vi "Measurement Logic.vi"() -> ()   [LabVIEW 2024, in "Analog Tachometer.lvlib"]
uses:
  Analog Tachometer.lvlib
  <vilib>/Plug-In SDKs/Measurements/Measure Call Context/Measure Call Context.lvclass
  Measurement Results.ctl
  <vilib>/gRPC/Generated APIs/ni/protobuf/types/RPC Messages/ni_protobuf_types_DoubleXYData.ctl
  <extravilib>/ChannelInstances/Event Messenger-bool/Instantiate.vi
  <vilib>/gRPC/Generated APIs/ni/protobuf/types/ni.protobuf.types.lvlib
  <vilib>/addons/Sound and Vibration/Order Analysis/Tach Process/SoundVib_TachProcess.lvlib
  <vilib>/addons/Sound and Vibration/Order Analysis/Utility/SoundVib_OAUtility.lvlib
  <vilib>/addons/Sound and Vibration/Order Analysis/Utility/SubVIs/oa_Buffer Settings.ctl
  <resource>/objmgr/daqmx.rc
  <vilib>/addons/Sound and Vibration/Order Analysis/Utility/OAT Output Buffered Data (XY, 1 Chan).vi
  <vilib>/DAQmx/read.llb/DAQmx Read (Analog Wfm 1Chan NSamp).vi
  <vilib>/addons/Sound and Vibration/Order Analysis/Tach Process/OAT Analog Tacho Process (1 Tacho).vi
  <vilib>/DAQmx/create/channels.llb/DAQmx Create Channel (AI-Voltage-Basic).vi
  <vilib>/DAQmx/configure/timing.llb/DAQmx Timing (Sample Clock).vi
  Measurement Configuration.ctl
panel:
  out "measurement results":T1
  in  "measurement configuration":T3={"sample rate"=1.2, "channel"="Lorem ipsum dolor sit", "max voltage"=32.0, "IEPE current"=32.0, "coupling"=64, "pulse/rev"=64, "threshold"=-32.0, "hysteresis"=-32.0, "slope (Rising)"=0} {"slope (Rising)" items=["Rising", "Falling"]; "coupling" items=["AC"=10045, "DC"=10050, "GND"=10066]}
  out "measure call context out":refnum<class "Measure Call Context.lvclass">
  in  "measure call context in":refnum<class "Measure Call Context.lvclass">
  out "error out":errorcluster
  in  "error in":errorcluster
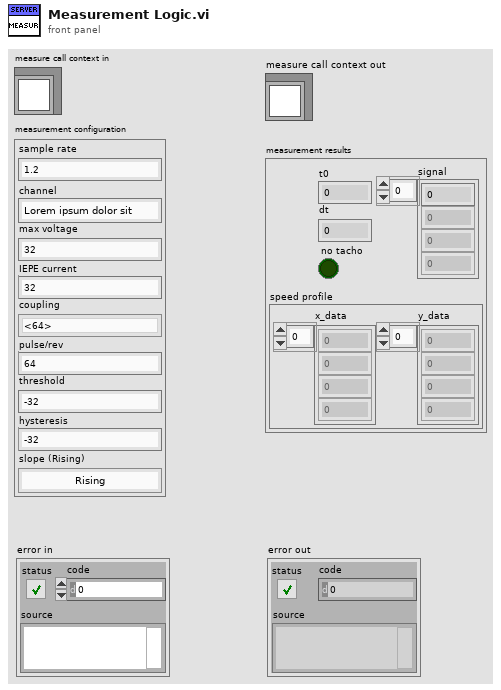
[diagram p1: front panel]
types:
  T1 = typedef "Analog Tachometer.lvlib/Measurement Results.ctl" = cluster{"t0":dbl, "dt":dbl, "signal":dbl[], "no tacho":bool, "speed profile":T2}
  T2 = typedef "ni.protobuf.types.lvlib/ni_protobuf_types_DoubleXYData.ctl" = cluster{"x_data":dbl[], "y_data":dbl[]}
  T3 = typedef "Analog Tachometer.lvlib/Measurement Configuration.ctl" = cluster{"sample rate":dbl, "channel":string, "max voltage":dbl, "IEPE current":dbl, "coupling":i32, "pulse/rev":i32, "threshold":dbl, "hysteresis":dbl, "slope (Rising)":u32}
  T4 = typedef "SoundVib_OAUtility.lvlib/oa_Buffer Settings.ctl" = cluster{"buffer size":dbl, "buffer unit":enum16{"s", "revolution", "# of samples"}}
  T5 = typedef "SoundVib_TachProcess.lvlib/speed profile.ctl" = cluster{"time [s]":dbl[], "speed [RPM]":dbl[]}
  T6 = typedef "OAT Position Info.ctl" = cluster{"positions [s]":dbl[], "samples/rev":dbl}
  T7 = typedef "Event Messenger-bool.lvlib/))Channel.ctl" = refnum<queue>
  T8 = typedef "Tag-bool.lvlib/))Channel.ctl" = refnum<queue>
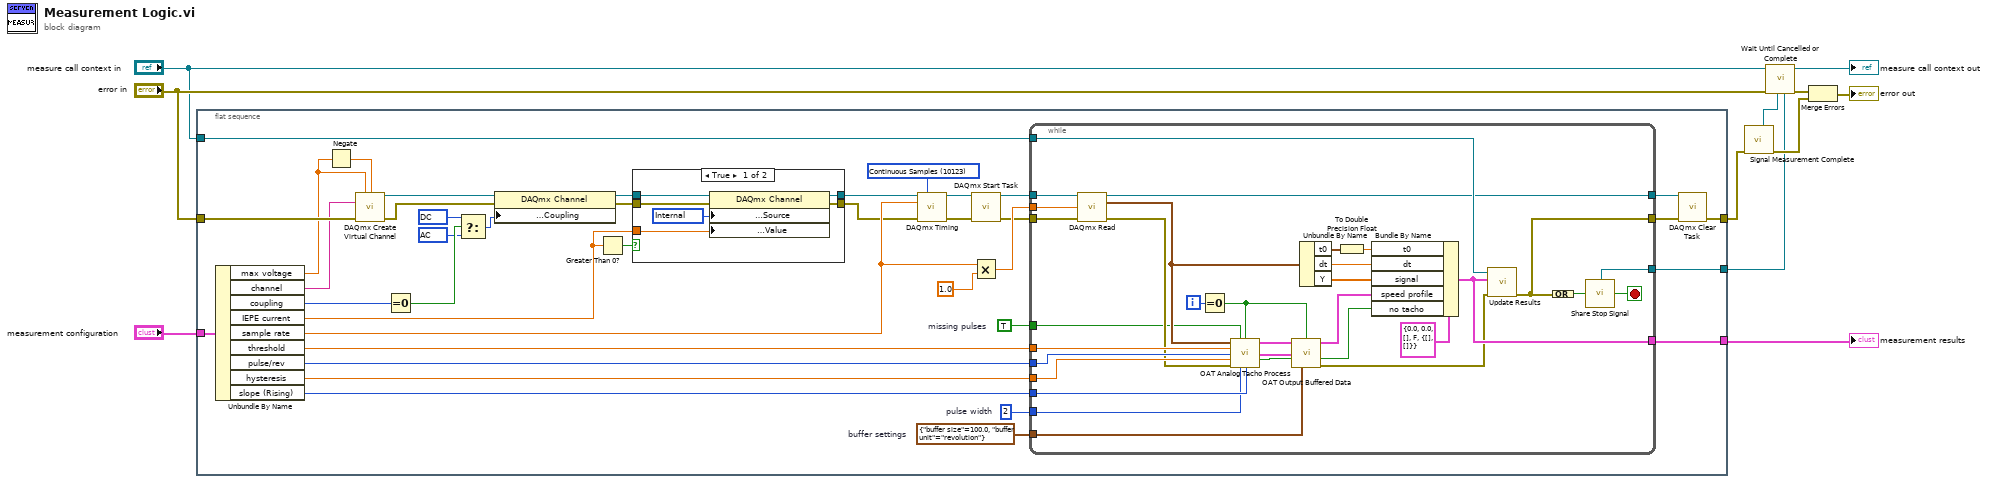
[diagram p0: block diagram]
diagram:
  n1 = flat-sequence {
    tunnel: "measurement configuration" -> [w50]
    tunnel: [w48] -> w10
    tunnel: "error in" -> [w31]
    tunnel: [w38] -> w7
    tunnel: w2 -> [w42]
    tunnel: "measure call context in" -> [w49]
    frame #0 {
      w12 = TRUE  # missing pulses
      w13 = 2  # pulse width
      w14 = T4 {"buffer size"=100.0, "buffer unit"=enum."revolution"}  # buffer settings
      w28 = 10045 items=["AC"=10045, "DC"=10050, "GND"=10066] ("AI.Coupling")
      w27 = 10050 items=["AC"=10045, "DC"=10050, "GND"=10066] ("AI.Coupling")
      w36 = 10123 items=["Finite Samples"=10178, "Continuous Samples"=10123, "Hardware Timed Single Point"=12522] ("sample mode")
      n2 = Unbundle By Name(w50) -> ("max voltage"=w20:dbl, "channel"=w21:string, "coupling"=w26:i32, "IEPE current"=w15:dbl, "sample rate"=w32:dbl, "threshold"=w45:dbl, "pulse/rev"=w44:i32, "hysteresis"=w43:dbl, "slope (Rising)"=w41:u32)
      n3 = Negate(x=w20) -> (-x=w19:dbl)
      n4 = call-poly <vilib>:"DAQmx Create Virtual Channel.vi"("maximum value"=w20, "minimum value"=w19, "physical channels"=w21, "error in"=w31) -> ("task out"=w17:refnum<k21>, "error out"=w18:errorcluster)  [unwired: 10 in]
      n5 = Equal To 0?(x=w26) -> (x = 0?=w29:bool)
      n6 = Select(t=w27, s=w29, f=w28) -> (s? t:f=w30:i32)
      n7 = property class="DAQmx Channel"(reference=w17, error in=w18, "Analog Input:General Properties:Input Configuration:Coupling"=w30) -> (reference out=w25:refnum<k21>, error out=w24:errorcluster)
      n8 = Greater Than 0?(x=w15) -> (x > 0?=w16:bool)
      n9 = case shown="True" w16 {
        tunnel: w25 -> [w86 w89]
        tunnel: w24 -> [w84 w88]
        tunnel: [w85 w89] -> w22
        tunnel: [w83 w88] -> w23
        tunnel: w15 -> [w82 _]
        frame True {
          w87 = 10200 items=["Internal"=10200, "External"=10167, "None"=10230] ("AI.Excit.Src")
          n10 = property class="DAQmx Channel"(reference=w86, error in=w84, "Analog Input:General Properties:Signal Conditioning:Excitation:Source"=w87, "Analog Input:General Properties:Signal Conditioning:Excitation:Value"=w82) -> (reference out=w85:refnum<k21>, error out=w83:errorcluster)
        }
        frame False {
        }
      }
      n11 = call-poly <vilib>:"DAQmx Timing.vi"("task/channels in"=w22, "sample mode"=w36, "rate"=w32, "error in"=w23) -> ("task out"=w37:refnum<k21>, "error out"=w35:errorcluster)  [unwired: 10 in]
      n12 = call <vilib>:"DAQmx Start Task.vi"("task/channels in"=w37, "error in"=w35) -> ("task out"=w34:refnum<k21>, "error out"=w33:errorcluster)  [unwired: 12 in]
      n13 = Multiply(x=w32, y=1.0) -> (x*y=w46:dbl)
      n14 = while {
        tunnel: w49 -> [w80]
        tunnel: [w79] -> w48
        tunnel: w46 -> [w78]
        tunnel: w45 -> [w77]
        tunnel: w44 -> [w76]
        tunnel: w43 -> [w75]
        tunnel: w42 -> [w62]
        tunnel: [w60] -> w39
        tunnel: w41 -> [w59]
        tunnel: [w58] -> w40
        tunnel: w34 -> [w55]
        tunnel: w33 -> [w54]
        tunnel: w14 -> [w53]
        tunnel: w13 -> [w52]
        tunnel: w12 -> [w51]
        i -> [w57]
        stop <- w63 stop-if-true
        n15 = call-poly <vilib>:"DAQmx Read.vi"("task/channels in"=w55, "number of samples per channel"=w78, "error in"=w54) -> ("task out"=w58:refnum<k21>, "data"=w72:waveform(dbl), "error out"=w65:errorcluster)  [unwired: 10 in]
        n16 = Equal To 0?(x=w57) -> (x = 0?=w56:bool)
        n17 = call-poly <vilib>:"OAT Analog Tacho Process.vi"("analog tacho signal"=w72, "missing pulses? (no:F)"=w51, "reset? (F)"=w56, "threshold (auto)"=w77, "pulse/revolution (1)"=w76, "hysteresis (0)"=w75, "error in (no error)"=w65, "pulse width (2)"=w52, "slope (Rising)"=w59) -> ("speed profile"=w73:T5, "speed position info"=w74:T6, "no tacho?"=w66:bool)  [unwired: 2 in, 2 out]
        n18 = call-poly <vilib>:"OAT Output Buffered Data.vi"("XY signal"=w73, "reset? (F)"=w56, "position info"=w74, "buffer settings"=w53) -> ("buffered XY signal"=w67:cluster{"X":dbl[], "Y":dbl[]}, "error out"=w64:errorcluster)  [unwired: 9 in, 1 out]
        n19 = Unbundle By Name(w72) -> ("t0"=w71:timestamp, "dt"=w69:dbl, "Y"=w68:dbl[])
        n20 = To Double Precision Float(number=w71) -> (double precision float=w70:dbl)
        n21 = Bundle By Name(cluster=T1 {"t0"=0.0, "dt"=0.0, "signal"=[], "no tacho"=FALSE, "speed profile"={"x_data"=[], "y_data"=[]}} ("Measurement Results"), "t0"=w70, "dt"=w69, "signal"=w68, "speed profile"=w67, "no tacho"=w66) -> (w79:T1)
        n22 = call <vilib>:"Update Results.vi"("error in"=w64, "measurement results"=w79, "measure call context in"=w80) -> ("error out"=w60:errorcluster)  [unwired: 7 in, 1 out]
        n23 = Compound Arithmetic op=OR(w60) -> (w61:bool)
        n24 = call <vilib>:"Share Stop Signal.vi"("set stop (F)"=w61, "channel"=w62) -> ("stop"=w63:bool)
      }
      n25 = call <vilib>:"DAQmx Clear Task.vi"("task in"=w40, "error in"=w39) -> ("error out"=w38:errorcluster)  [unwired: 13 in]
    }
  }
  n26 = call "Signal Measurement Complete.vi"("error in (no error)"=w7) -> ("error out"=w5:errorcluster, "done channel"=w6:T7)  [unwired: 9 in]
  n27 = call "Wait Until Cancelled or Complete.vi"("done channel"=w6, "error in (no error)"="error in", "measure call context in"="measure call context in") -> ("error out"=w4:errorcluster, "measure call context out"=→"measure call context out":refnum<class "Measure Call Context.lvclass">, "stop channel"=w2:T8)  [unwired: 6 in]
  n28 = Merge Errors(w4, w5) -> (→"error out":errorcluster)
  "measurement results" <- w10
